vi "Clear Registered Paths.vi"(8 "error in (no error)":errorcluster) -> (0 "error out":errorcluster, 3 "Cleared Paths":path[](array[path]))   [LabVIEW 2021, in "Path Utilities.lvlib"]
doc: "Clear all registered paths. Deleted paths are listed in Cleared Paths array.\n\nNo error is returned."
uses:
  Path Utilities.lvlib
  TypeDefs/FGV State - Path Registration.ctl
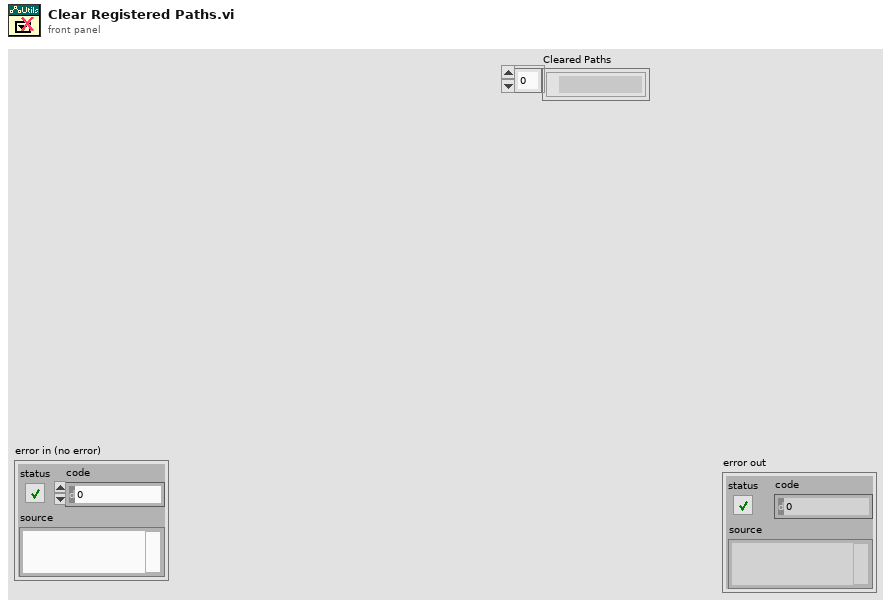
[diagram p1: front panel]
types:
  T1 = typedef "Path Utilities.lvlib/FGV State - Path Registration.ctl" = enum16{"Get Path", "List All Paths", "Register Path", "Unregister Path", "Empty Map"}
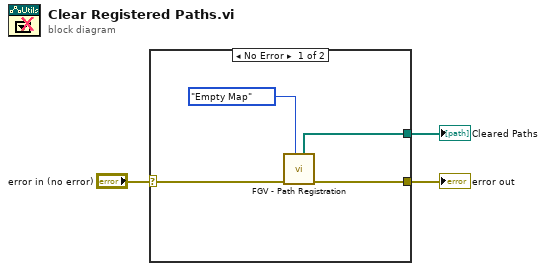
[diagram p0: block diagram]
diagram:
  n1 = case shown="No Error" "error in (no error)" {
    selector: "error in (no error)" -> [w7 w8]
    tunnel: [w6 w8] -> w2
    tunnel: [w4 _] -> w1
    frame No Error {
      n2 = call "FGV - Path Registration.vi"("FGV State"=FGV_State_-_Path_Registration."Empty Map", "error in (no error)"=w7) -> ("error out"=w6:errorcluster, "All Paths"=w4:path[])  [unwired: 4 in, 4 out]
    }
    frame Error {
    }
  }
  "error out" <- w2
  "Cleared Paths" <- w1
